vi "Max Current to Integer.vi"(11 "Current (mA)":dbl) -> (3 "Current Int":i16)   [LabVIEW 2016, in "Laser Diode Controller.lvlib" / "KLD101.lvclass"]
uses:
  KLD101.lvclass
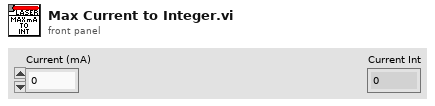
[diagram p1: front panel]
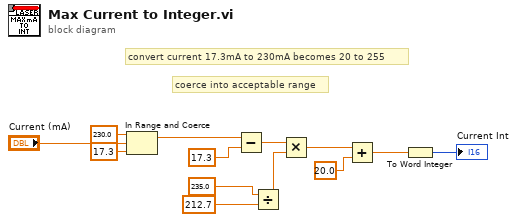
[diagram p0: block diagram]
diagram:
  # "coerce into acceptable range"
  # "convert current 17.3mA to 230mA becomes 20 to 255"
  n1 = In Range and Coerce(upper limit=230.0, x="Current (mA)", lower limit=17.3) -> (coerced(x)=w3:dbl)  [unwired: 1 out]
  n2 = Subtract(x=w3, y=17.3) -> (x-y=w9:dbl)
  n3 = Divide(x=235.0 ("y"), y=212.7) -> (x/y=w7:dbl)
  n4 = Multiply(x=w9, y=w7) -> (x*y=w8:dbl)
  n5 = Add(x=w8, y=20.0) -> (x+y=w10:dbl)
  n6 = To Word Integer(number=w10) -> (16bit integer=→"Current Int":i16)
